vi "calcoloTransizioniSubVi.vi"(0 "Array":dbl[](array[numeric])=array[616821 elements]) -> (1 "indice di inizio":i32[](array[numeric])=[0, 0, 0, 0, 0, 1, 1, 1, 1, 1, 1, 1, 1, 1, 1, 1, 1, 1, 2, 2, 2, 2, 2, 2, 2, 2, 2, 2, 2, 2, 2, 3, 3, 3, 3, 3, 3, 3, 3, 3, 3, 3, 3, 4, 4, 4, 4, 4, 4, 4, 4, 4, 4, 4, 4, 4, 5, 5, 5, 5, 5, 5, 5, 5, 5, 5, 5, 5, 5, 6, 6, 6, 6, 6, 6, 6, 6, 6, 6, 6, 6, 6, 7, 7, 7, 7, 7, 7, 7, 7, 7, 7, 7, 7, 8, 8, 8, 8, 8, 8, 8, 8, 8, 8, 8, 8, 8, 9, 9, 9, 9, 9, 9, 9, 9, 9, 9, 9, 9, 9, 10, 10, 10, 10, 10, 10, 10, 10, 10, 10, 10, 10, 10, 11, 11, 11, 11, 11, 11, 11, 11, 11, 11, 11, 11, 11, 12, 12, 12, 12, 12, 12, 12, 12, 12, 12, 12, 12, 12, 13, 13, 13, 13, 13, 13, 13, 13, 13, 13, 13, 13, 14, 14, 14, 14, 14, 14, 14, 14, 14, 14, 14, 14, 14, 15, 15, 15, 15, 15, 15, 15, 15, 15, 15, 15, 15, 15, 16, 16, 16, 16, 16, 16, 16, 16, 16, 16, 16, 16, 16, 17, 17, 17, 17, 17, 17, 17, 17, 17, 17, 17, 17, 18, 18, 18, 18, 18, 18, 18, 18, 18, 18, 18, 18, 18, 19, 19, 19, 19, 19, 19, 19, 19, 19, 19, 19], 2 "indice di fine":i32[](array[numeric])=[0, 0, 0, 0, 0, 1, 1, 1, 1, 1, 1, 1, 1, 1, 1, 1, 1, 1, 2, 2, 2, 2, 2, 2, 2, 2, 2, 2, 2, 2, 2, 3, 3, 3, 3, 3, 3, 3, 3, 3, 3, 3, 3, 4, 4, 4, 4, 4, 4, 4, 4, 4, 4, 4, 4, 4, 5, 5, 5, 5, 5, 5, 5, 5, 5, 5, 5, 5, 5, 6, 6, 6, 6, 6, 6, 6, 6, 6, 6, 6, 6, 6, 7, 7, 7, 7, 7, 7, 7, 7, 7, 7, 7, 7, 8, 8, 8, 8, 8, 8, 8, 8, 8, 8, 8, 8, 8, 9, 9, 9, 9, 9, 9, 9, 9, 9, 9, 9, 9, 9, 10, 10, 10, 10, 10, 10, 10, 10, 10, 10, 10, 10, 10, 11, 11, 11, 11, 11, 11, 11, 11, 11, 11, 11, 11, 11, 12, 12, 12, 12, 12, 12, 12, 12, 12, 12, 12, 12, 12, 13, 13, 13, 13, 13, 13, 13, 13, 13, 13, 13, 13, 14, 14, 14, 14, 14, 14, 14, 14, 14, 14, 14, 14, 14, 15, 15, 15, 15, 15, 15, 15, 15, 15, 15, 15, 15, 15, 16, 16, 16, 16, 16, 16, 16, 16, 16, 16, 16, 16, 16, 17, 17, 17, 17, 17, 17, 17, 17, 17, 17, 17, 17, 18, 18, 18, 18, 18, 18, 18, 18, 18, 18, 18, 18, 18, 19, 19, 19, 19, 19, 19, 19, 19, 19, 19, 19])   [LabVIEW 2018]
panel:
  out "size(s) 2":i32
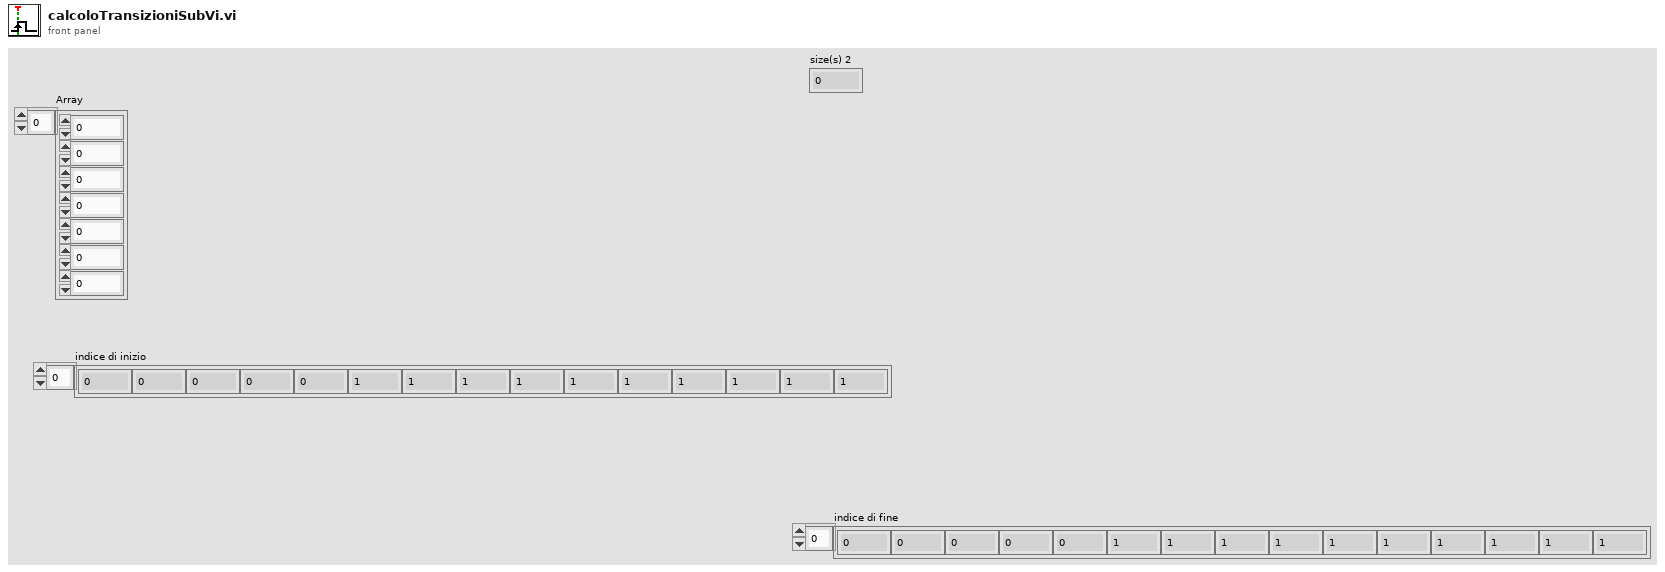
[diagram p1: front panel]
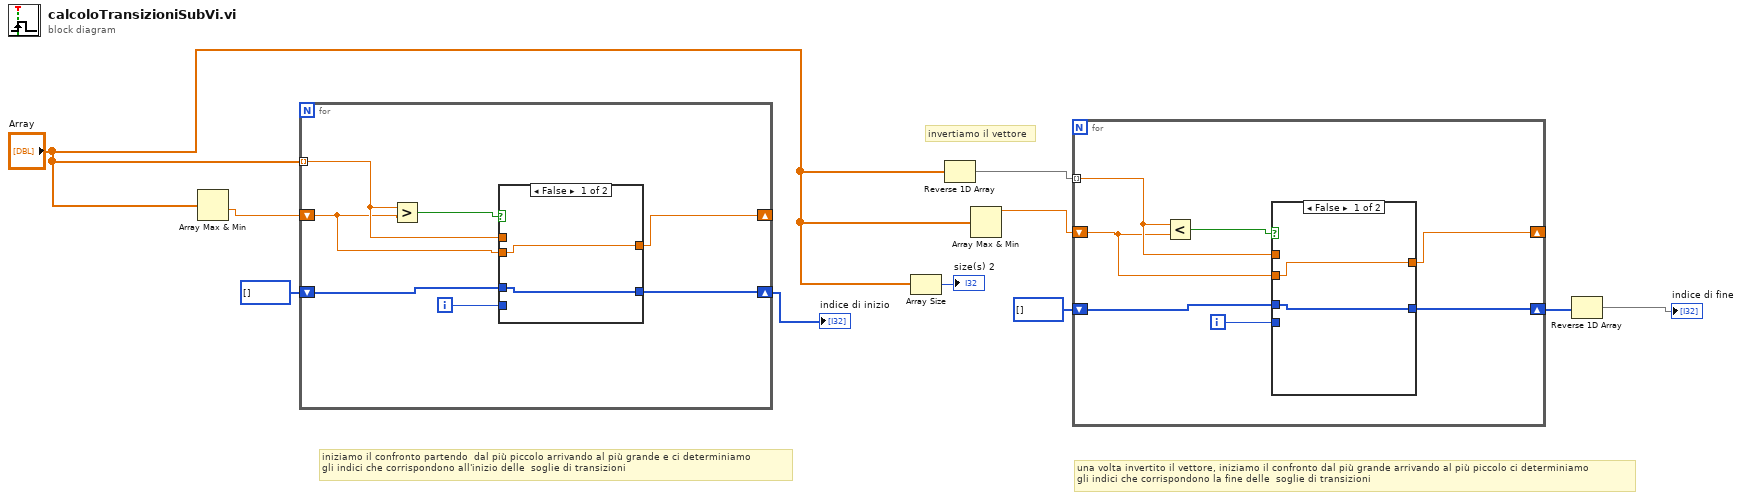
[diagram p0: block diagram]
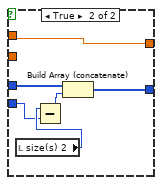
[diagram p2: hidden frame]
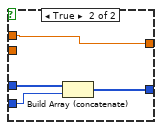
[diagram p3: hidden frame]
diagram:
  # "una volta invertito il vettore, iniziamo il confronto dal più grande arrivando al più piccolo ci determiniamo\ngli indici che corrispondono la fine delle  soglie di transizioni"
  # "invertiamo il vettore"
  # "iniziamo il confronto partendo  dal più piccolo arrivando al più grande e ci determiniamo\ngli indici che corrispondono all'inizio delle  soglie di transizioni"
  n1 = Array Max & Min(array="Array") -> (min value=w2:dbl)  [unwired: 3 out]
  n2 = for {
    shift-right: [w13] -> _
    shift-left: w2 -> [w11]
    tunnel: "Array" -> [w12] mode=indexing
    shift-right: [w14] -> w4
    shift-left: i32[] [] -> [w15]
    i -> [w16]
    n3 = Greater?(x=w12, y=w11) -> (0:w17:bool)
    n4 = case shown="False" w17 {
      tunnel: w12 -> [_ w20]
      tunnel: w16 -> [_ w23]
      tunnel: w15 -> [w19 w22]
      tunnel: [w19 w21] -> w14
      tunnel: [w18 w20] -> w13
      tunnel: w11 -> [w18 _]
      frame False {
      }
      frame True {
        n5 = Build Array (concatenate)(w22, w23) -> (w21:i32[])
      }
    }
  }
  "indice di inizio" <- w4
  n6 = Array Size(array="Array") -> (size(s)=→"size(s) 2":i32)
  n7 = Reverse 1D Array(array="Array") -> (reversed array=w7:dbl[])
  n8 = Array Max & Min(array="Array") -> (max value=w6:dbl)  [unwired: 3 out]
  n9 = for {
    shift-right: [w26] -> _
    shift-left: w6 -> [w24]
    tunnel: w7 -> [w25] mode=indexing
    shift-right: [w27] -> w9
    shift-left: i32[] [] -> [w28]
    i -> [w29]
    n10 = Less?(x=w25, y=w24) -> (x < y?=w30:bool)
    n11 = case shown="False" w30 {
      tunnel: w25 -> [_ w33]
      tunnel: w29 -> [_ w35]
      tunnel: w28 -> [w32 w38]
      tunnel: [w32 w37] -> w27
      tunnel: [w31 w33] -> w26
      tunnel: w24 -> [w31 _]
      frame False {
      }
      frame True {
        n12 = local read "size(s) 2"() -> (w36:i32)
        n13 = Subtract(x=w36, y=w35) -> (x-y=w34:i32)
        n14 = Build Array (concatenate)(w38, w34) -> (w37:i32[])
      }
    }
  }
  n15 = Reverse 1D Array(array=w9) -> (reversed array=→"indice di fine":i32[])
